vi "IMAQdx Serial Read Bytes.vi"(7 "Timeout (ms)":u32=1000, 8 "error in":errorcluster, 10 "Bytes to Read":u32, 11 "Session In":T1) -> (0 "error out":errorcluster, 1 "Bytes Read":u32, 2 "Data Bytes":u8[](array[numeric]), 3 "Session Out":T1)   [LabVIEW 2020, in "NI_Vision_Acquisition_Software.lvlib"]
doc: "Reads in an expected number of bytes from the serial port on image acquisition devices that support serial communication."
uses:
  NI_Vision_Acquisition_Software.lvlib
  IMAQdx.ctl
  niimaqdx.dll
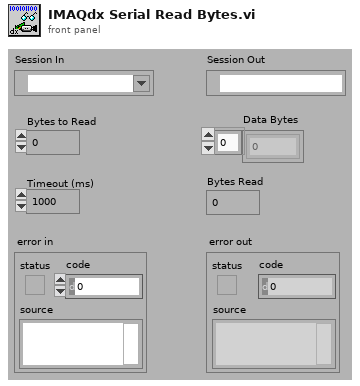
[diagram p1: front panel]
types:
  T1 = typedef "IMAQdx.ctl" = refnum<k21>
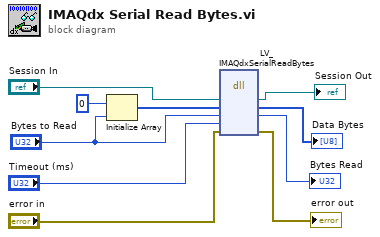
[diagram p0: block diagram]
diagram:
  n1 = Initialize Array(u8 0 ("element"), "Bytes to Read") -> (w5:u8[])
  n2 = dll-call lib="niimaqdx.dll" fn="LV_IMAQdxSerialReadBytes"("refnum"="Session In", "buffer"=w5, "bufferSize"="Bytes to Read", "timeOut"="Timeout (ms)", "error"="error in") -> ("refnum"=→"Session Out":T1, "buffer"=→"Data Bytes":u8[], "bufferSize"=→"Bytes Read":u32, "error"=→"error out":errorcluster)  [unwired: 4 in, 3 out]
